vi "sdp810-csv-to-data.vi"(10 "sensor-name":string, 11 "sensor-csv-input":string) -> (1 "SDP810: Temp (degC)":dbl format="%.2f", 2 "SDP810: diff Pressure (mBar)":dbl format="%.2f", 3 "SDP810: data output":T1 {"Humidity (%)" format="%.2f"; "Temp (degC)" format="%.2f"})   [LabVIEW 2021]
uses:
  SHT41.ctl
  SDP810.ctl
  <vilib>/regexp/Match Regular Expression.xnode
panel:
  out "SDP810: Temperature":string
  out "SDP810: diff Pressure":string
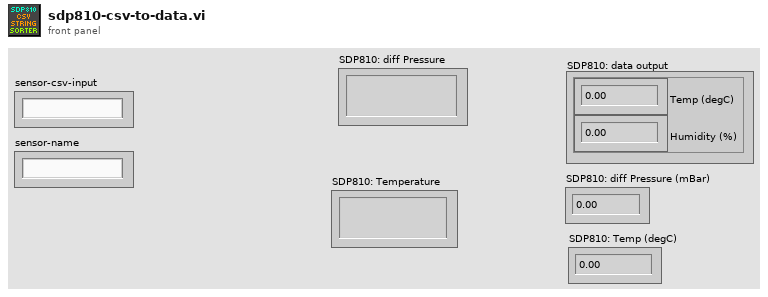
[diagram p1: front panel]
types:
  T1 = typedef "SHT41.ctl" = cluster{"Temp (degC)":dbl, "Humidity (%)":dbl}
  T2 = typedef "SDP810.ctl" = cluster{"dP (mBar)":dbl, "Temp (degC)":dbl}
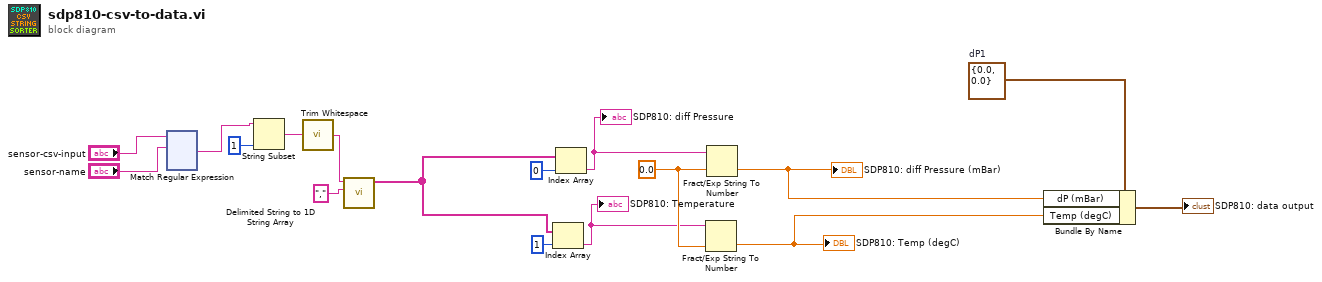
[diagram p0: block diagram]
diagram:
  w14 = T2 {"dP (mBar)"=0.0, "Temp (degC)"=0.0}  # dP1
  w17 = 0.0
  n1 = xnode "Match Regular Expression"("input string"="sensor-csv-input", "regular expression"="sensor-name") -> ("after match"=w1:string)  [unwired: 4 in, 4 out]
  n2 = String Subset(string=w1, offset (0)=1) -> (substring=w2:string)  [unwired: 1 in]
  n3 = call <vilib>:"Trim Whitespace.vi"("string"=w2) -> ("trimmed string"=w12:string)  [unwired: 1 in]
  n4 = call <vilib>:"Delimited String to 1D String Array.vi"("delimiter"=",", "delimited string"=w12) -> ("string array"=w6:string[])  [unwired: 9 in]
  n5 = Index Array(array=w6, index=1) -> (element=w4:string)
  "SDP810: Temperature" <- w4
  n6 = Index Array "Index Array"(array=w6, index=0) -> (element=w5:string)
  "SDP810: diff Pressure" <- w5
  n7 = Fract/Exp String To Number(string=w4, default (0 dbl)=w17) -> (number=w15:dbl)  [unwired: 2 in, 1 out]
  "SDP810: Temp (degC)" <- w15
  n8 = Fract/Exp String To Number(string=w5, default (0 dbl)=w17) -> (number=w16:dbl)  [unwired: 2 in, 1 out]
  "SDP810: diff Pressure (mBar)" <- w16
  n9 = Bundle By Name(cluster=w14, "dP (mBar)"=w16, "Temp (degC)"=w15) -> (→"SDP810: data output":T2)
